vi "运维调试_总磷总氮.vi"() -> ()   [LabVIEW 2016, in "斯坦道CODcr.lvlib"]
uses:
  <vilib>/Utility/miscctls.llb/LVPointTypeDef.ctl
  <vilib>/Plasmionique/MB Master/MB_Master/MB_Master.lvclass
  <vilib>/ptbypt/NI_PtbyPt.lvlib
panel:
  out "seconds since 1Jan1904 2":timestamp
  out "seconds since 1Jan1904":timestamp
  in  "周期设置":bool
  in  "流程操作":bool
  out "消解压力":sgl format="%#.2f kPa"
  out "权限等级":string
  out "总步数":i32
  out "滑动杆":u8(slide) caption="测试进度" scale=0.0..100.0
  out "试剂余量显示":sgl[][](graph)
  in  "仪器校准":bool
  in  "参数查询":bool
  out "简易步骤名称":string
  in  "温度曲线":bool
  in  "试剂余量":bool
  in  "灯值调整":bool
  out "固件版本号":string
  out "模块版本号":string
  out "注射器温度":sgl format="%#.2f ℃"
  out "消解温度":sgl format="%#.2f ℃"
  out "ADC":sgl
  out "F3":sgl format="%#.6f"
  out "F2":sgl format="%#.6f"
  out "F1":sgl format="%#.6f"
  out "F0":sgl format="%#.6f"
  out "运行状态":T1 {"数据时间:" format="%<%y/%m/%d %H:%M:%S>T"; "仪器时间:" format="%<%y/%m/%d %H:%M:%S>T"}
  in  "单选按钮":T2=enum."总氮"
  in  "布尔":bool
  in  "外设固件":bool
  out "字符串 2":string
  in  "数组":string[](array[string])
  in  "返回":bool
  in  "参数设置":bool
  out "集成报警信息":string
  in  "停止":bool
  in  "手动启动":bool
  in  "调试":bool
  out "多列列表框":i32(listbox)
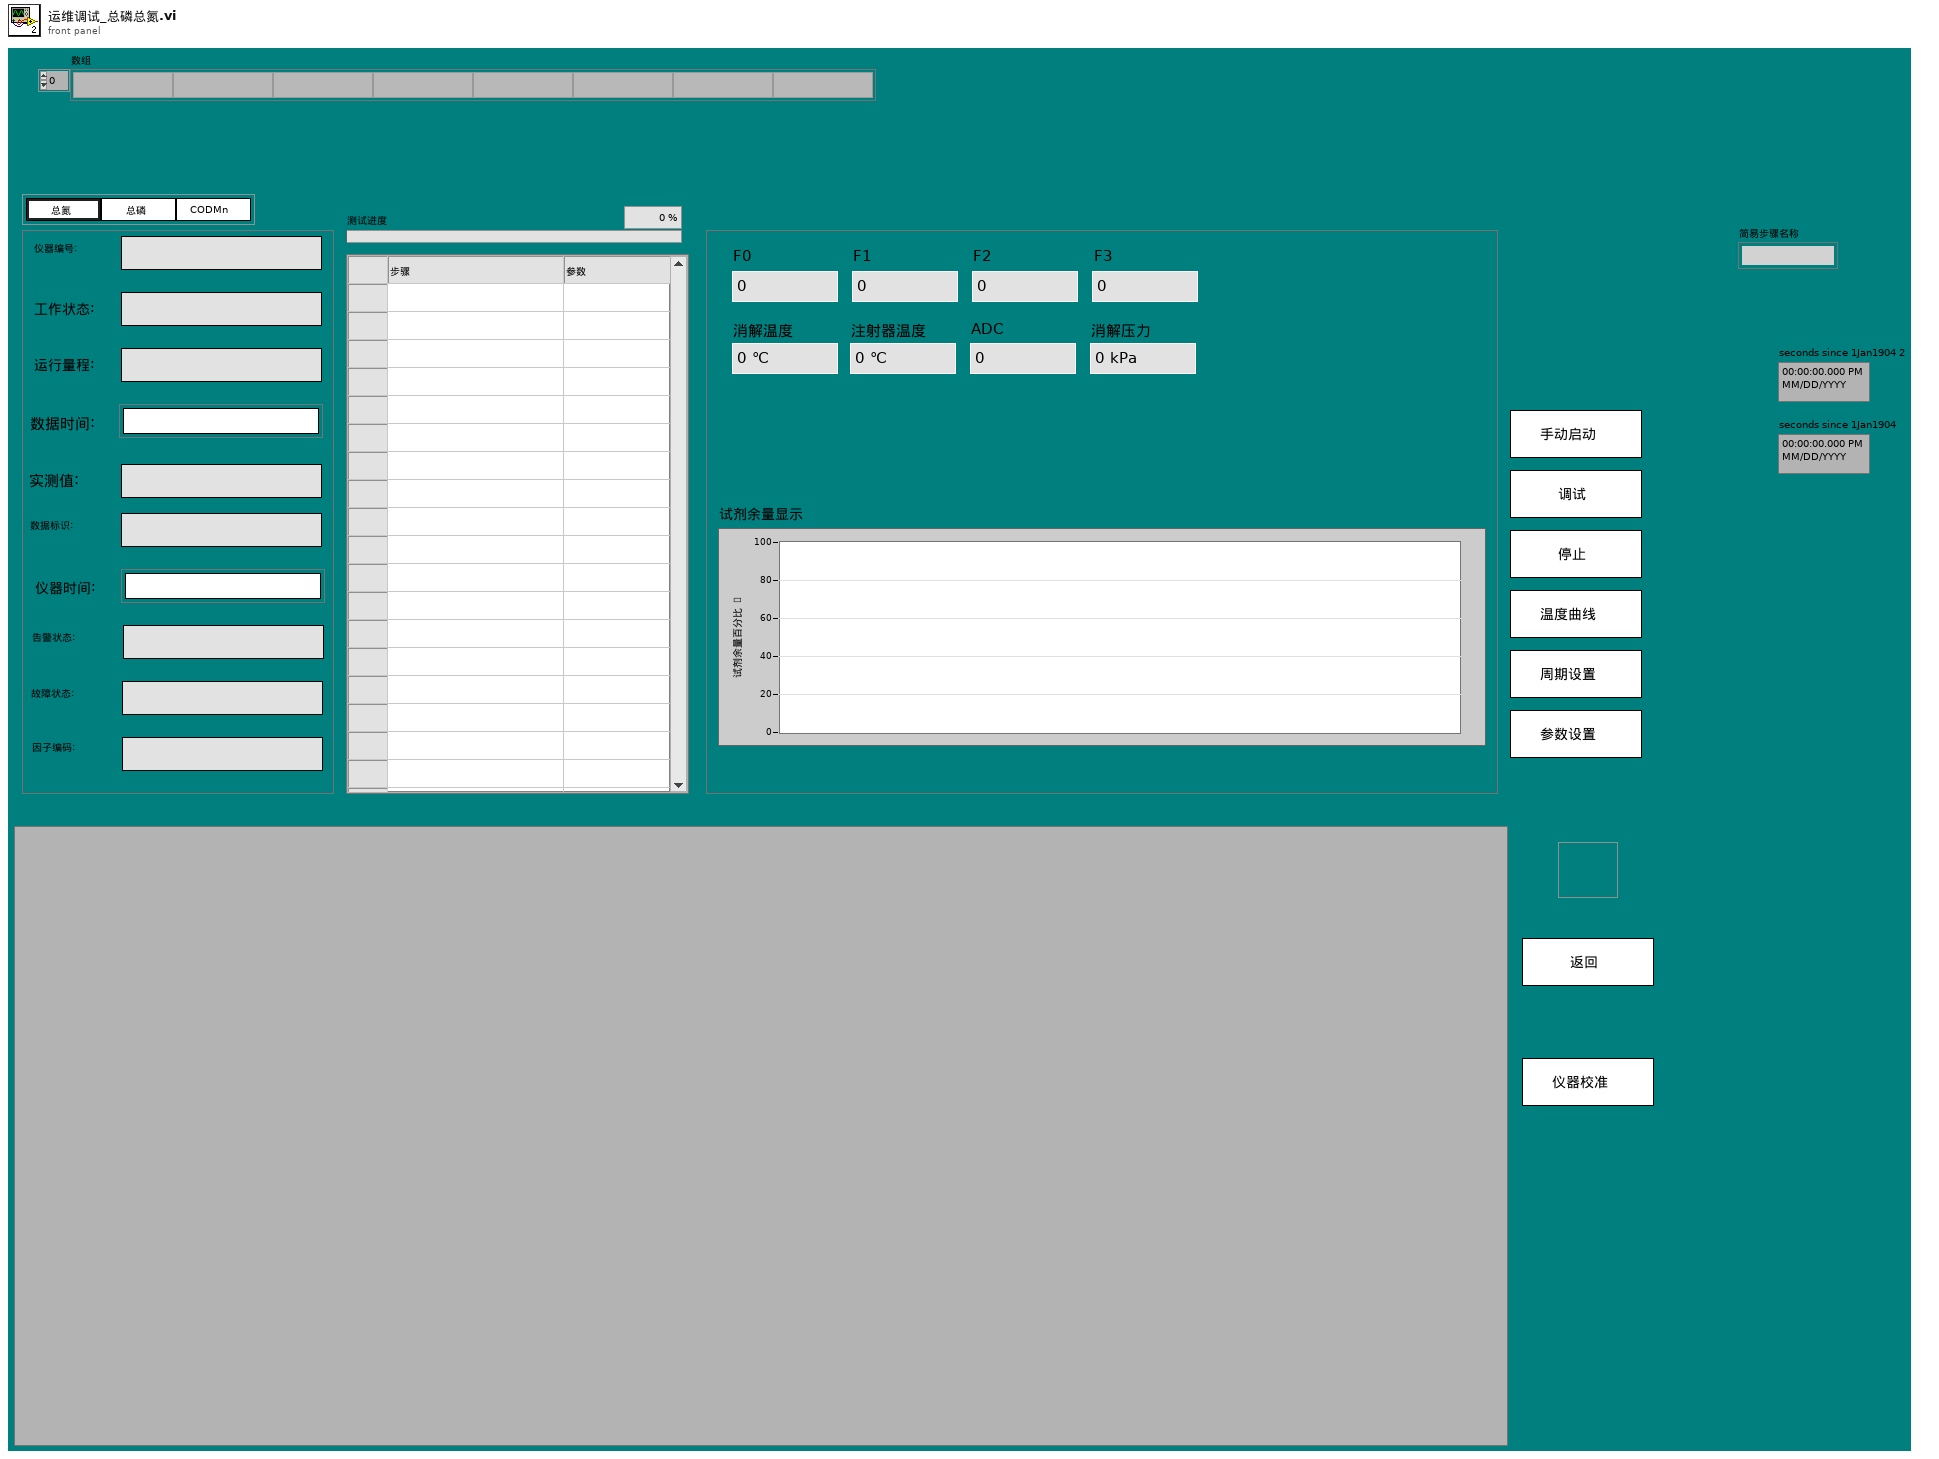
[diagram p1: front panel]
types:
  T1 = cluster{"仪器编号:":string, "工作状态:":string, "运行量程: ":string, "数据时间:":timestamp, "实测值:":string, "数据标识: ":string, "仪器时间:":timestamp, "告警状态: ":string, "故障状态:  ":string, "因子编码:":string}
  T2 = typedef "斯坦道CODcr.lvlib/启动参数显示控件.ctl" = enum32{"COD", "氨氮", "总氮", "总磷", "磷酸盐", "硝氮", "亚硝氮", "硅酸盐", "硫化物", "氟化物", "CODMn"}
  T3 = cluster{"Major":u16, "Minor":u16, "Fix":u16, "Build":u16}
  T4 = typedef "斯坦道总磷总氮.lvlib/启动参数显示控件.ctl" = enum32{"COD", "氨氮", "总氮", "总磷", "磷酸盐", "硝氮", "亚硝氮", "硅酸盐", "硫化物", "氟化物", "CODMn"}
  T5 = typedef "LVPointTypeDef.ctl" = cluster{"Horizontal":i16, "Vertical":i16}
  T6 = cluster{"系统时间":timestamp, "工作状态":u16, "测量模式":enum16{"待机", "连续模式", "周期模式", "定点模式", "受控模式", "手动模式"}, "告警代码":u16, "故障代码":u16, "日志代码":u16, "软件版本":u16, "F0":sgl, "F1":sgl, "F2":sgl, "F3":sgl, "T":sgl, "H":sgl, "id":u16, "flowid":u16, "量程":u16, "总磷控温温度1":sgl, "营养盐控温温度2":sgl, "ADC":sgl}
  T7 = cluster{"id":string, "ver":string, "type":string, "code":u16, "level":enum16{"一级", "二级", "三级"}, "message":string, "analysis":string, "platform_alarm_code":string}
  T8 = typedef "SingleStepTestV3.lvlib/SingleStepTestV3.lvclass/仪器版本.ctl" = enum16{"A版", "B版", "A1版"}
  T9 = cluster{"因子编码":u32, "单位":u16, "标样参考值":sgl, "水样数据时间":timestamp, "水样实测值":sgl, "水样数据标识":string, "标样数据时间":timestamp, "标样实测值":sgl, "标样数据标识":string, "空白数据时间":timestamp, "空白实测值":sgl, "空白数据标识":string, "零点核查数据时间":timestamp, "零点核查实测值":sgl, "零点核查数据标识":string, "跨度核查数据时间":timestamp, "跨度核查实测值":sgl, "跨度核查数据标识":string, "加标回收数据时间":timestamp, "加标回收实测值":sgl, "加标回收数据标识":string, "平行样数据时间":timestamp, "平行样实测值":sgl, "平行样数据标识":string, "F0":sgl, "F1":sgl, "F2":sgl, "F3":sgl, "F4":sgl, "F5":sgl, "F6":sgl, "F7":sgl, "温度":sgl, "湿度":sgl, "X值":sgl, "fidrange":u16, "X1值":sgl}[]
  T10 = cluster{"因子编码":u32, "单位":u16, "标样参考值":sgl, "水样数据时间":timestamp, "水样实测值":sgl, "水样数据标识":string, "标样数据时间":timestamp, "标样实测值":sgl, "标样数据标识":string, "空白数据时间":timestamp, "空白实测值":sgl, "空白数据标识":string, "零点核查数据时间":timestamp, "零点核查实测值":sgl, "零点核查数据标识":string, "跨度核查数据时间":timestamp, "跨度核查实测值":sgl, "跨度核查数据标识":string, "加标回收数据时间":timestamp, "加标回收实测值":sgl, "加标回收数据标识":string, "平行样数据时间":timestamp, "平行样实测值":sgl, "平行样数据标识":string, "F0":sgl, "F1":sgl, "F2":sgl, "F3":sgl, "F4":sgl, "F5":sgl, "F6":sgl, "F7":sgl, "温度":sgl, "湿度":sgl, "X值":sgl, "fidrange":u16, "X1值":sgl}
  T11 = typedef "报警信息字段定义.ctl" = cluster{"时间":timestamp, "参数":string, "报警信息":string, "备注":string, "code":u64, "platform_alarm_code":string, "报警标识":enum16{"产生", "消除"}}
  T12 = typedef "TimingControl.lvlib/TimingControl.lvclass/国标控制命令.ctl" = enum16{"启动测量", "标样核查", "零点核查", "跨度核查", "空白测试", "平行样测试", "加标回收", "空白校准", "标样校准", "初始化（清洗）", "停止测试", "仪器重启", "校时", "模式设置", "测量间隔设置"}
  T13 = typedef "TimingControl.lvlib/TimingControl.lvclass/测量参数.ctl" = u16
  T14 = enum32{"Bad", "Idle", "Run top level", "Running"}
  T15 = enum16{"空闲", "水样测试", "标样核查", "零点核查", "跨度核查", "空白测试", "平行样测试", "加标回收", "空白校准", "标样校准", "初始化（清洗）"}
  T16 = cluster{"站号":u16, "量程切换":enum32{"H", "L", "AUTO"}, "控制命令":enum16{"启动测量", "标样核查", "零点核查", "跨度核查", "空白测试", "平行样测试", "加标回收", "空白校准", "标样校准", "初始化（清洗）", "停止测试", "仪器重启", "校时", "模式设置", "测量间隔设置"}, "模式设置":enum16{"待机", "连续模式", "周期模式", "定点模式", "受控模式", "手动模式"}, "测量间隔":u16}
  T17 = cluster{"时间标识":timestamp, "设备":string, "日志信息":string, "流程参数":string}
  T18 = typedef "LVRowAndColumnUnsignedTypeDef.ctl" = cluster{"Row":u32, "Column":u32}
  T19 = typedef "操作日志字段定义.ctl" = cluster{"时间":timestamp, "参数":string, "日志信息":string, "流程参数":string}
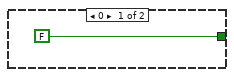
[diagram p4: hidden frame]
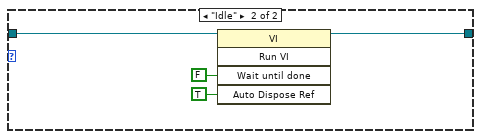
[diagram p8: hidden frame]
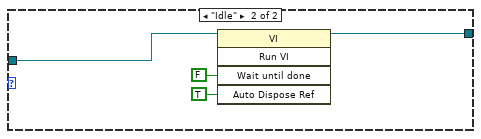
[diagram p9: hidden frame]
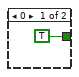
[diagram p11: hidden frame]
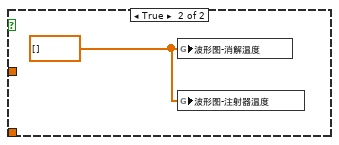
[diagram p12: hidden frame]
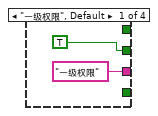
[diagram p18: hidden frame]
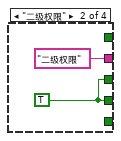
[diagram p19: hidden frame]
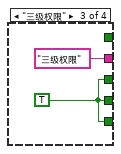
[diagram p20: hidden frame]
diagram:
  n1 = flat-sequence {
    tunnel: [w28] -> w18
    tunnel: w18 -> [w40]
    tunnel: [w40] -> w17
    tunnel: w17 -> [w65]
    tunnel: [w156] -> w19
    tunnel: [errorcluster {"status"=FALSE, "code"=0, "source"=""} ("错误输入（无错误）")] -> w8
    tunnel: [errorcluster {"status"=FALSE, "code"=0, "source"=""} ("错误输入（无错误）")] -> w7
    tunnel: [w153] -> w5
    tunnel: [errorcluster {"status"=FALSE, "code"=0, "source"=""} ("error out")] -> w4
    tunnel: [errorcluster {"status"=FALSE, "code"=0, "source"=""} ("错误输入（无错误）")] -> w3
    frame #0 {
      n2 = control-ref of="本VI"() -> (w30:refnum<vi>)
      n3 = control-ref of="本VI"() -> (w39:refnum<vi>)
      n4 = property class="VI"(reference=w30) -> ("Library"=w31:refnum<vi>)  [unwired: 1 in, 2 out]
      n5 = property class="VI"(reference=w39) -> ("Library.Version"=w38:T3)  [unwired: 1 in, 2 out]
      n6 = global read "VAR总磷总氮全局变量.vi" "初始化"() -> (w27:bool)
      n7 = case shown="假" w27 {
        frame False {
          n8 = call "配置初始化.vi"() -> ()  [unwired: 11 in, 1 out]
        }
        frame True {
        }
      }
      n9 = property class="Library"(reference=w31) -> ("Path"=w29:path)  [unwired: 1 in, 2 out]
      n10 = Unbundle By Name(w38) -> ("Major"=w36:u16, "Minor"=w35:u16, "Fix"=w34:u16, "Build"=w33:u16)
      n11 = call "新建通讯互斥锁.vi"() -> ()  [unwired: 11 in, 1 out]
      n12 = Format Into String(format string="模块版本号：%d.%d.%d.%d" ("格式字符串"), w36, w35, w34, w33) -> (resulting string=→"模块版本号":string)  [unwired: 2 in, 1 out]
      n13 = call <vilib>:"Get File Extension.vi"("file"=w29) -> ("filename without extension"=w28:string)  [unwired: 6 in, 4 out]
    }
    frame #1 {
      n14 = global read "总磷总氮断电保存全局变量.vi" "IP"() -> (w44:string)
      n15 = global read "总磷总氮断电保存全局变量.vi" "VISA Resource"() -> (w41:refnum<visa-resource-name>)
      n16 = Empty String/Path?(string/path=w44) -> (empty?=w43:bool)
      n17 = Empty String/Path?(string/path=w41) -> (empty?=w42:bool)
      n18 = case shown="真" w43 {
        tunnel: w40 -> [_ w56]
        frame False {
        }
        frame True {
          n19 = case shown="\"斯坦道CODMn\"" w56 {
            tunnel: [w57 "192.168.1.203" ("IP") "192.168.1.202" ("IP") "192.168.1.202" ("IP") "192.168.1.203" ("IP") "192.168.1.204" ("IP") "192.168.1.205" ("IP") "192.168.1.201" ("IP")] -> w55
            frame Default {
              n20 = global read "总磷总氮断电保存全局变量.vi" "IP"() -> (w57:string)
            }
            frame "斯坦道总磷总氮" {
            }
            frame "斯坦道氨氮" {
            }
            frame "斯坦道氨氮总磷" {
            }
            frame "斯坦道总磷" {
            }
            frame "斯坦道总氮" {
            }
            frame "斯坦道CODcr" {
            }
            frame "斯坦道CODMn" {
            }
          }
          n21 = global write "总磷总氮断电保存全局变量.vi" "IP"(w55) -> ()
        }
      }
      n22 = case shown="真" w42 {
        tunnel: w40 -> [_ w46]
        frame False {
        }
        frame True {
          n23 = case shown="\"斯坦道CODMn\"" w46 {
            tunnel: [w47 "COM5" ("IP") "COM7" ("IP") "COM7" ("IP") "COM5" ("IP") "COM10" ("IP") "COM9" ("IP") "COM4" ("IP")] -> w45
            frame Default {
              n24 = global read "总磷总氮断电保存全局变量.vi" "VISA Resource"() -> (w47:refnum<visa-resource-name>)
            }
            frame "斯坦道总磷总氮" {
            }
            frame "斯坦道氨氮" {
            }
            frame "斯坦道氨氮总磷" {
            }
            frame "斯坦道总磷" {
            }
            frame "斯坦道总氮" {
            }
            frame "斯坦道CODcr" {
            }
            frame "斯坦道CODMn" {
            }
          }
          n25 = global write "总磷总氮断电保存全局变量.vi" "VISA Resource"(w45) -> ()
        }
      }
    }
    frame #2 {
      n26 = global read "model config var.vi" "启动队列名称"() -> (w67:cluster{"String":string, "Value":u16}[])
      n27 = Empty Array?(array=w67) -> (empty?=w66:bool)
      n28 = case shown="真" w66 {
        tunnel: w65 -> [_ w68]
        frame False {
        }
        frame True {
          n29 = global read "总磷总氮断电保存全局变量.vi" "PORT"() -> (w74:string)
          n30 = Decimal String To Number(string=w74) -> (number=w73:i32)  [unwired: 2 in, 1 out]
          n31 = global read "总磷总氮断电保存全局变量.vi" "MB通信方式选择"() -> (w72:enum16{"串口", "TCP"})
          n32 = global read "总磷总氮断电保存全局变量.vi" "VISA Resource"() -> (w71:refnum<visa-resource-name>)
          n33 = global read "总磷总氮断电保存全局变量.vi" "IP"() -> (w75:string)
          n34 = call "获取启动参数.vi"("MB通信方式选择"=w72, "Port (502)"=w73, "IP Address"=w75, "VISA Resource"=w71) -> ("error out"=w70:errorcluster, "数组"=w69:cluster{"String":string, "Value":u16}[])  [unwired: 6 in]
          n35 = flat-sequence {
            tunnel: w70 -> [w77]
            tunnel: w69 -> [w76]
            tunnel: w68 -> [w79]
            frame #0 {
              n36 = case shown="无错误" w77 {
                tunnel: w76 -> [w78 _]
                frame No Error {
                  n37 = global write "model config var.vi" "启动队列名称"(w78) -> ()
                }
                frame Error {
                }
              }
            }
            frame #1 {
              n38 = global read "model config var.vi" "启动队列名称"() -> (w81:cluster{"String":string, "Value":u16}[])
              n39 = Empty Array?(array=w81) -> (empty?=w80:bool)
              n40 = case shown="真" w80 {
                tunnel: w79 -> [_ w82]
                frame False {
                }
                frame True {
                  n41 = case shown="\"斯坦道CODmn\"" w82 {
                    frame Default {
                    }
                    frame "斯坦道总磷总氮" {
                      n42 = global write "model config var.vi" "启动队列名称"(cluster{"String":string, "Value":u16}[] [{"String"="总氮", "Value"=2}, {"String"="总磷", "Value"=1}] ("启动队列名称")) -> ()
                    }
                    frame "斯坦道氨氮" {
                      n43 = global write "model config var.vi" "启动队列名称"(cluster{"String":string, "Value":u16}[] [{"String"="氨氮", "Value"=3}] ("启动队列名称")) -> ()
                    }
                    frame "斯坦道氨氮总磷" {
                      n44 = global write "model config var.vi" "启动队列名称"(cluster{"String":string, "Value":u16}[] [{"String"="氨氮", "Value"=3}, {"String"="总磷", "Value"=1}] ("启动队列名称")) -> ()
                    }
                    frame "斯坦道总磷" {
                      n45 = global write "model config var.vi" "启动队列名称"(cluster{"String":string, "Value":u16}[] [{"String"="总磷", "Value"=1}] ("启动队列名称")) -> ()
                    }
                    frame "斯坦道总氮" {
                      n46 = global write "model config var.vi" "启动队列名称"(cluster{"String":string, "Value":u16}[] [{"String"="总氮", "Value"=2}] ("启动队列名称")) -> ()
                    }
                    frame "斯坦道CODcr" {
                      n47 = global write "model config var.vi" "启动队列名称"(cluster{"String":string, "Value":u16}[] [{"String"="CODcr", "Value"=22}] ("启动队列名称")) -> ()
                    }
                    frame "斯坦道氟化物" {
                      n48 = global write "model config var.vi" "启动队列名称"(cluster{"String":string, "Value":u16}[] [{"String"="氟化物", "Value"=50}] ("启动队列名称")) -> ()
                    }
                    frame "斯坦道CODmn" {
                      n49 = global write "model config var.vi" "启动队列名称"(cluster{"String":string, "Value":u16}[] [{"String"="CODMn", "Value"=21}] ("启动队列名称")) -> ()
                    }
                  }
                }
              }
            }
            frame #2 {
              n50 = call "模块配置写入.vi"() -> ()  [unwired: 11 in, 1 out]
            }
          }
        }
      }
    }
    frame #3 {
      # "初始化"
      n51 = global read "总磷总氮断电保存全局变量.vi" "流程路径"() -> (w95:path)
      n52 = global read "model config var.vi" "启动队列名称"() -> (w101:cluster{"String":string, "Value":u16}[])
      n53 = global read "总磷总氮断电保存全局变量.vi" "简易流程路径"() -> (w92:path)
      n54 = call <vilib>:"Check if File or Folder Exists.vi"("path"=w95) -> ("file or folder exists?"=w100:bool)  [unwired: 8 in, 2 out]
      n55 = for {
        tunnel: w101 -> [w118] mode=indexing
        shift-right: [w117] -> w102
        shift-left: "" -> [w115]
        n56 = Unbundle By Name(w118) -> ("String"=w116:string)
        n57 = Concatenate Strings(w115, w116) -> (w117:string)
      }
      n58 = call <vilib>:"Check if File or Folder Exists.vi"("path"=w92) -> ("file or folder exists?"=w99:bool)  [unwired: 8 in, 2 out]
      n59 = Empty String/Path?(string/path=w95) -> (empty?=w96:bool)
      n60 = Not(x=w100) -> (.not. x?=w98:bool)
      n61 = Empty String/Path?(string/path=w92) -> (empty?=w91:bool)
      n62 = Not(x=w99) -> (.not. x?=w94:bool)
      n63 = Or(x=w96, y=w98) -> (x .or. y?=w97:bool)
      n64 = Or(x=w91, y=w94) -> (x .or. y?=w93:bool)
      n65 = case shown="真" w97 {
        frame False {
        }
        frame True {
          n66 = global read "model config var.vi" "启动队列名称"() -> (w111:cluster{"String":string, "Value":u16}[])
          n67 = for {
            tunnel: w111 -> [w114] mode=indexing
            tunnel: [w113] -> w110 mode=indexing
            n68 = Unbundle By Name(w114) -> ("String"=w113:string)
          }
          n69 = call "获取默认流程路径.vi"("参数"=w110) -> ("路径"=w112:path)  [unwired: 10 in]
          n70 = global write "总磷总氮断电保存全局变量.vi" "流程路径"(w112) -> ()
        }
      }
      n71 = case shown="真" w93 {
        frame False {
        }
        frame True {
          n72 = global read "model config var.vi" "启动队列名称"() -> (w106:cluster{"String":string, "Value":u16}[])
          n73 = for {
            tunnel: w106 -> [w109] mode=indexing
            tunnel: [w108] -> w105 mode=indexing
            n74 = Unbundle By Name(w109) -> ("String"=w108:string)
          }
          n75 = call "获取默认流程路径.vi"("复合步骤"=TRUE, "参数"=w105) -> ("路径"=w107:path)  [unwired: 9 in]
          n76 = global write "总磷总氮断电保存全局变量.vi" "简易流程路径"(w107) -> ()
        }
      }
      n77 = global write "VAR总磷总氮全局变量.vi" "模块名称"(w102) -> ()
    }
    frame #4 {
      n78 = global read "model config var.vi" "启动队列名称"() -> (w121:cluster{"String":string, "Value":u16}[])
      n79 = vi-ref "总磷总氮测量数据储存.vi"() -> (w131:refnum<vi>)
      n80 = vi-ref "总磷总氮通讯.vi"() -> (w123:refnum<vi>)
      n81 = Index Array(array=w121) -> (element=w120:cluster{"String":string, "Value":u16})  [unwired: 1 in]
      n82 = property class="VI"(reference=w131) -> ("Name"=w138:string)  [unwired: 1 in, 2 out]
      n83 = property class="VI"(reference=w123) -> ("Name"=w124:string)  [unwired: 1 in, 2 out]
      n84 = Unbundle By Name(w120) -> ("Value"=w119:u16)
      n85 = case shown="50" w119 {
        tunnel: [w139 启动参数显示控件."总磷" ("单选按钮") 启动参数显示控件."总氮" ("单选按钮") 启动参数显示控件."COD" ("单选按钮") 启动参数显示控件."氨氮" ("单选按钮") 启动参数显示控件."磷酸盐" ("单选按钮") 启动参数显示控件."硝氮" ("单选按钮") 启动参数显示控件."亚硝氮" ("单选按钮") 启动参数显示控件."硅酸盐" ("单选按钮") 启动参数显示控件."硫化物" ("单选按钮") 启动参数显示控件."氟化物" ("单选按钮") 启动参数显示控件."CODMn" ("单选按钮")] -> w122
        frame 0, Default {
          n86 = property on="单选按钮" class="RadioBtnsControl (严格)"() -> ("Value"=w139:T4)  [unwired: 2 in, 2 out]
        }
        frame 1 {
        }
        frame 2 {
        }
        frame 22 {
        }
        frame 3 {
        }
        frame 4 {
        }
        frame 5 {
        }
        frame 6 {
        }
        frame 7 {
        }
        frame 8 {
        }
        frame 50 {
        }
        frame 21 {
        }
      }
      n87 = Open VI Reference(type specifier VI Refnum (for type only)=refnum<vi> refnum, vi path=w138, options=128 ("选项")) -> (vi reference=w136:refnum<vi>, error out=w134:errorcluster)  [unwired: 3 in]
      n88 = Open VI Reference(type specifier VI Refnum (for type only)=refnum<vi> refnum, vi path=w124, options=128 ("选项")) -> (vi reference=w126:refnum<vi>, error out=w128:errorcluster)  [unwired: 3 in]
      n89 = call-by-ref "开始异步调用"(reference=w136, error in=w134) -> (reference out=w132:refnum<vi>, error out=w133:errorcluster)  [unwired: 12 in]
      n90 = call-by-ref "开始异步调用"(reference=w126, error in=w128) -> (reference out=w130:refnum<vi>, error out=w129:errorcluster)  [unwired: 12 in]
      n91 = Close Reference(reference=w132, error in (no error)=w133) -> ()  [unwired: 1 out]
      n92 = Close Reference(reference=w130, error in (no error)=w129) -> ()  [unwired: 1 out]
      n93 = property on="单选按钮" class="RadioBtnsControl (严格)"("Value"=w122) -> ()  [unwired: 2 in, 2 out]
    }
    frame #5 {
      n94 = call "配置文件路径.vi"() -> ("appended path"=w153:path)  [unwired: 11 in]
      n95 = call "设置模块队列名.vi"() -> ("Msg"=w156:string)  [unwired: 5 in]
    }
  }
  n96 = flat-sequence {
    frame #0 {
      n97 = property on="窗格" class="Pane"("Origin"=T5 {"Horizontal"=0, "Vertical"=0} ("原点")) -> ()  [unwired: 2 in, 2 out]
    }
  }
  n98 = call "Create balloon 队列.vi"() -> ("队列输出"=w23:refnum<queue>)  [unwired: 11 in]
  n99 = while {
    stop <- FALSE stop-if-true
    n100 = global read "VAR总磷总氮全局变量.vi" "状态告警区"() -> (w162:T6)
    n101 = Unbundle By Name(w162) -> ("工作状态"=w160:u16)
    n102 = Equal To 0?(x=w160) -> (x = 0?=w159:bool)
    n103 = global read "VAR总磷总氮全局变量.vi" "通讯状态"() -> (w163:bool)
    n104 = And(x=w159, y=w163) -> (x .and. y?=w161:bool)
    n105 = call <vilib>:"Boolean Crossing PtByPt.vi"("input"=w161) -> ("crossing"=w158:bool)  [unwired: 2 in]
    n106 = case shown="真" w158 {
      frame False {
      }
      frame True {
        n107 = control-ref of="试剂余量显示"() -> (w166:refnum<vi>)
        n108 = call "试剂余量展示.vi"("波形图 2"=w166) -> ("波形图"=→"试剂余量显示":sgl[][])  [unwired: 10 in]
      }
    }
    n109 = Wait (ms)(milliseconds to wait=u32 1000 ("等待时间（毫秒）")) -> ()  [unwired: 1 out]
  }
  n110 = while {
    shift-right: [w177] -> _
    shift-left: u32 0 ("y") -> [w179]
    stop <- FALSE stop-if-true
    # "密码权限"
    n111 = global read "VAR总磷总氮全局变量.vi" "权限等级"() -> (w174:enum16{"一级权限", "二级权限", "三级权限", "超级权限"})
    n112 = case shown="\"超级权限\"" w174 {
      tunnel: [_ w184 w186 w189] -> w168
      tunnel: [_ _ w186 w189] -> _
      tunnel: [_ w184 w186 w189] -> w173
      tunnel: [_ _ _ TRUE] -> _
      tunnel: [TRUE _ _ _] -> w171
      tunnel: ["一级权限" "二级权限" "三级权限" "超级权限"] -> w169
      frame "一级权限", Default {
      }
      frame "二级权限" {
        w184 = TRUE
      }
      frame "三级权限" {
        w186 = TRUE
      }
      frame "超级权限" {
        w189 = TRUE
      }
    }
    "权限等级" <- w169
    n113 = case shown="假" "布尔" {
      tunnel: w179 -> [_ w192]
      tunnel: [_ w191] -> w177
      frame False {
      }
      frame True {
        n114 = Increment(x=w192) -> (x+1=w191:u32)
      }
    }
    n115 = Wait (ms)(milliseconds to wait=u32 1000 ("等待时间（毫秒）")) -> ()  [unwired: 1 out]
    n116 = Not(x=w171) -> (.not. x?=w170:bool)
    n117 = property on="外设固件" class="Bool"("Visible"=w173) -> ()  [unwired: 2 in, 2 out]
    n118 = property on="流程操作" class="Bool"("Visible"=w168) -> ()  [unwired: 2 in, 2 out]
    n119 = property on="试剂余量" class="Bool"("Visible"=w168) -> ()  [unwired: 2 in, 2 out]
    n120 = property on="灯值调整" class="Bool"("Visible"=w168) -> ()  [unwired: 2 in, 2 out]
    n121 = Greater Or Equal?(x=w177, y=u32 3600) -> (x >= y?=w175:bool)
    n122 = property on="布尔" class="Bool (严格)"("Value"=w170) -> ()  [unwired: 2 in, 2 out]
    n123 = case shown="真" w175 {
      frame False {
      }
      frame True {
        n124 = global write "VAR总磷总氮全局变量.vi" "权限等级"(enum16{"一级权限", "二级权限", "三级权限", "超级权限"}."一级权限" ("权限等级")) -> ()
      }
    }
  }
  n125 = while {
    shift-right: [w203] -> _
    shift-left: u16 1 ("工作状态") -> [w201]
    stop <- FALSE stop-if-true
    (unwired) "注射器温度"
    n126 = global read "VAR总磷总氮全局变量.vi" "状态告警区"() -> (w224:T6)
    n127 = global read "VAR总磷总氮全局变量.vi" "通讯状态"() -> (w235:bool)
    n128 = global read "VAR总磷总氮全局变量.vi" "状态告警区"() -> (w233:T6)
    n129 = global write "VAR总磷总氮全局变量.vi" "最近一次工作状态"(w201) -> ()
    n130 = Unbundle By Name(w224) -> ("id"=w223:u16, "工作状态"=w219:u16)
    n131 = case shown="真" w235 {
      tunnel: ["通讯异常" ("集成报警信息") w354] -> w234
      frame False {
      }
      frame True {
        n132 = global read "VAR总磷总氮全局变量.vi" "状态告警区"() -> (w356:T6)
        n133 = local read "seconds since 1Jan1904 2"() -> (w346:timestamp)
        n134 = local read "seconds since 1Jan1904"() -> (w349:timestamp)
        n135 = Subtract(x=w346, y=w349) -> (x-y=w345:dbl)
        n136 = Unbundle By Name(w356) -> ("工作状态"=w352:u16)
        n137 = Not Equal To 0?(x=w352) -> (x != 0?=w348:bool)
        n138 = Get Date/Time In Seconds() -> (seconds since 1Jan1904=w347:timestamp)
        n139 = global read "VAR总磷总氮全局变量.vi" "测量状态"() -> (w353:string)
        n140 = Greater Or Equal?(x=w345, y=36000.0) -> (x >= y?=w342:bool)
        n141 = case shown="真" w348 {
          tunnel: w347 -> [_ w357]
          frame False {
          }
          frame True {
            "seconds since 1Jan1904 2" <- w357
          }
        }
        n142 = Format Into String(format string="工作计时: %d 秒" ("格式字符串"), initial string=w353, w345) -> (resulting string=w354:string)  [unwired: 1 in, 1 out]
        n143 = call <vilib>:"Boolean Crossing PtByPt.vi"("direction"=enum16{"either", "false-true", "true-false"}."false-true", "input"=w348) -> ("crossing"=w350:bool)  [unwired: 1 in]
        n144 = Or(x=w350, y=w342) -> (x .or. y?=w343:bool)
        n145 = case shown="真" w343 {
          tunnel: w347 -> [_ w358]
          frame False {
          }
          frame True {
            "seconds since 1Jan1904" <- w358
          }
        }
      }
    }
    "集成报警信息" <- w234
    n146 = Unbundle By Name(w233) -> ("flowid"=w200:u16, "系统时间"=w229:timestamp, "工作状态"=w228:u16, "告警代码"=w222:u16, "故障代码"=w221:u16, "量程"=w227:u16)
    n147 = case shown="\"磷酸盐\"" "单选按钮" {
      tunnel: [22 3 2 1 4 5 6 7 8 50 21] -> w204
      tunnel: [_ TRUE _ _ _ _ _ _ _ _ _] -> w195
      frame "COD", Default {
      }
      frame "氨氮" {
      }
      frame "总氮" {
      }
      frame "总磷" {
      }
      frame "磷酸盐" {
      }
      frame "硝氮" {
      }
      frame "亚硝氮" {
      }
      frame "硅酸盐" {
      }
      frame "硫化物" {
      }
      frame "氟化物" {
      }
      frame "CODMn" {
      }
    }
    n148 = case shown="1, 默认" w219 {
      tunnel: w223 -> [_ w291]
      frame 0 {
      }
      frame 1, Default {
        n149 = case shown="21" w291 {
          tunnel: [w292 启动参数显示控件."总磷" ("单选按钮") 启动参数显示控件."总氮" ("单选按钮") 启动参数显示控件."COD" ("单选按钮") 启动参数显示控件."氨氮" ("单选按钮") 启动参数显示控件."磷酸盐" ("单选按钮") 启动参数显示控件."硝氮" ("单选按钮") 启动参数显示控件."亚硝氮" ("单选按钮") 启动参数显示控件."硅酸盐" ("单选按钮") 启动参数显示控件."硫化物" ("单选按钮") 启动参数显示控件."CODMn" ("单选按钮") 启动参数显示控件."氟化物" ("单选按钮")] -> w290
          frame 0, Default {
            n150 = property on="单选按钮" class="RadioBtnsControl (严格)"() -> ("Value"=w292:T4)  [unwired: 2 in, 2 out]
          }
          frame 1 {
          }
          frame 2 {
          }
          frame 22 {
          }
          frame 3 {
          }
          frame 4 {
          }
          frame 5 {
          }
          frame 6 {
          }
          frame 7 {
          }
          frame 8 {
          }
          frame 21 {
          }
          frame 50 {
          }
        }
        n151 = property on="单选按钮" class="RadioBtnsControl (严格)"("Value"=w290) -> ()  [unwired: 2 in, 2 out]
      }
    }
    n152 = case shown="2" w228 {
      selector: w228 -> [w308 _ w314 w318 w321 w323 w325 w327 w329 w331 w333 w335 w337 w340]
      tunnel: [w309 "空闲" ("工作状态") "水样测量" ("工作状态") w317 "零点核查" ("工作状态") "跨度核查" ("工作状态") "空白测试" ("工作状态") "平行样测试" ("工作状态") "加标回收" ("工作状态") "空白校准" ("工作状态") "标样校准" ("工作状态") "初始化" ("工作状态") "单步调试" ("工作状态") w339] -> w202
      tunnel: [w307 w312 w314 w318 w321 w323 w325 w327 w329 w331 w333 w335 w337 w340] -> w203
      tunnel: w201 -> [w307 w312 _ _ _ _ _ _ _ _ _ _ _ _]
      tunnel: w200 -> [_ _ _ w316 _ _ _ _ _ _ _ _ _ _]
      frame Default {
        n153 = Format Into String(format string="%d" ("格式字符串"), initial string="未知" ("工作状态"), w308) -> (resulting string=w309:string)  [unwired: 1 in, 1 out]
      }
      frame 0 {
      }
      frame 1 {
      }
      frame 2 {
        n154 = case shown="5" w316 {
          tunnel: ["标样核查" ("工作状态") "快捷测试" ("工作状态")] -> w317
          frame 0, Default {
          }
          frame 5 {
          }
        }
      }
      frame 3 {
      }
      frame 4 {
      }
      frame 5 {
      }
      frame 6 {
      }
      frame 7 {
      }
      frame 8 {
      }
      frame 9 {
      }
      frame 10 {
      }
      frame 254 {
      }
      frame 255 {
        n155 = local read "简易步骤名称"() -> (w339:string)
      }
    }
    n156 = call "告警码字段定义.vi"("告警代码"=w222) -> ("告警信息"=w199:T7)  [unwired: 10 in]
    n157 = call "故障码字段定义.vi"("故障代码"=w221) -> ("告警信息"=w220:T7)  [unwired: 10 in]
    n158 = case shown="1" w227 {
      tunnel: ["" ("字符串") "低量程 " ("字符串") "高量程 " ("字符串")] -> w226
      frame Default {
      }
      frame 0 {
      }
      frame 1 {
      }
    }
    n159 = Unbundle By Name(w199) -> ("message"=w198:string)
    n160 = Unbundle By Name(w220) -> ("message"=w193:string)
    n161 = call "id参数转换.vi"("id"=w204) -> ("数组资源索引"=w205:i32)  [unwired: 9 in, 1 out]
    n162 = call "版本判断.vi"() -> ("仪器版本"=w197:T8)  [unwired: 11 in]
    n163 = global read "VAR总磷总氮全局变量.vi" "测量数据区数组"() -> (w208:T9)
    n164 = case shown="\"A版\", 默认" w197 {
      tunnel: [w238 "传感器" ("标题.文本")] -> w194
      tunnel: ["%#.2f ℃" ("数值文本.格式字符串") "%#.2f " ("数值文本.格式字符串")] -> w196
      tunnel: w195 -> [w241 _]
      frame "A版", Default {
        n165 = Select(t="显色温度", s=w241, f="注射器温度" ("标题.文本")) -> (s? t:f=w238:string)
      }
      frame "B版" {
      }
    }
    n166 = Index Array(array=w208, index=w205) -> (element=w207:T10)
    n167 = case shown="0, 默认" w201 {
      tunnel: [w259 w265 w269 w273 w277 w281 w285 w289] -> w218
      tunnel: [w257 w264 w268 w272 w275 w280 w284 w288] -> w213
      tunnel: [w260 w263 w267 w271 w274 w279 w283 w287] -> w211
      tunnel: w207 -> [_ w262 w266 w270 w276 w278 w282 w286]
      frame 0, Default {
        n168 = local read "运行状态"() -> (w261:T1)
        n169 = Unbundle By Name(w261) -> ("数据时间:"=w259:timestamp, "实测值:"=w258:string, "数据标识:"=w260:string)
        n170 = Fract/Exp String To Number(string=w258) -> (number=w257:dbl)  [unwired: 3 in, 1 out]
      }
      frame 1 {
        n171 = Unbundle By Name(w262) -> ("水样数据时间"=w265:timestamp, "水样实测值"=w264:sgl, "水样数据标识"=w263:string)
      }
      frame 2, 9 {
        n172 = Unbundle By Name(w266) -> ("标样数据时间"=w269:timestamp, "标样实测值"=w268:sgl, "标样数据标识"=w267:string)
      }
      frame 3 {
        n173 = Unbundle By Name(w270) -> ("零点核查数据时间"=w273:timestamp, "零点核查实测值"=w272:sgl, "零点核查数据标识"=w271:string)
      }
      frame 4 {
        n174 = Unbundle By Name(w276) -> ("跨度核查数据时间"=w277:timestamp, "跨度核查实测值"=w275:sgl, "跨度核查数据标识"=w274:string)
      }
      frame 7 {
        n175 = Unbundle By Name(w278) -> ("加标回收数据时间"=w281:timestamp, "加标回收实测值"=w280:sgl, "加标回收数据标识"=w279:string)
      }
      frame 5, 8 {
        n176 = Unbundle By Name(w282) -> ("空白数据时间"=w285:timestamp, "空白实测值"=w284:sgl, "空白数据标识"=w283:string)
      }
      frame 6 {
        n177 = Unbundle By Name(w286) -> ("平行样数据时间"=w289:timestamp, "平行样实测值"=w288:sgl, "平行样数据标识"=w287:string)
      }
    }
    n178 = Unbundle By Name(w207) -> ("因子编码"=w209:u32)
    n179 = global write "VAR总磷总氮全局变量.vi" "工作状态:"(w202) -> ()
    n180 = Format Into String(format string="w%05d" ("格式字符串"), w209) -> (resulting string=w225:string)  [unwired: 2 in, 1 out]
    n181 = property on="注射器温度" class="DigNum (严格)"("Caption.Text"=w194, "NumText.FormatString"=w196) -> ()  [unwired: 2 in, 2 out]
    n182 = Wait (ms)(milliseconds to wait=u32 1000 ("等待时间（毫秒）")) -> ()  [unwired: 1 out]
    n183 = Number To Fractional String(number=w213, precision (6)=i16 4 ("精度(6)")) -> (F-format string=w215:string)  [unwired: 2 in]
    n184 = Concatenate Strings(w215, " " ("字符串"), "mg/L" ("字符串")) -> (w212:string)
    n185 = global read "VAR总磷总氮全局变量.vi" "序列号"() -> (w230:string)
    n186 = Bundle By Name(cluster=T1 {"仪器编号:"="", "工作状态:"="", "运行量程: "="", "数据时间:"=timestamp(0 s since 1904-01-01), "实测值:"="", "数据标识: "="", "仪器时间:"=timestamp(0 s since 1904-01-01), "告警状态: "="", "故障状态:  "="", "因子编码:"=""} ("运行状态"), "仪器编号:"=w230, "仪器时间:"=w229, "工作状态:"=w202, "告警状态:"=w198, "故障状态:"=w193, "运行量程:"=w226, "数据时间:"=w218, "实测值:"=w212, "数据标识:"=w211, "因子编码:"=w225) -> (→"运行状态":T1)
  }
  n187 = while {
    shift-right: [w363] -> _
    shift-left: 0 -> [w364]
    stop <- FALSE stop-if-true
    n188 = global read "VAR总磷总氮全局变量.vi" "心跳包打开状态"() -> (w359:bool)
    n189 = case shown="假" w359 {
      tunnel: w364 -> [w368 _]
      tunnel: [w367 _] -> w363
      frame False {
        n190 = Increment(x=w368) -> (x+1=w367:i32)
      }
      frame True {
      }
    }
    n191 = Wait (ms)(milliseconds to wait=u32 1000 ("等待时间（毫秒）")) -> ()  [unwired: 1 out]
    n192 = Greater Or Equal?(x=w363, y=600) -> (x >= y?=w361:bool)
    n193 = case shown="真" w361 {
      frame False {
      }
      frame True {
        n194 = global write "VAR总磷总氮全局变量.vi" "升级固件关闭心跳包"(FALSE ("关闭心跳包")) -> ()
      }
    }
  }
  n195 = while {
    shift-right: [w370] -> _
    shift-left: TRUE -> [w371]
    stop <- FALSE stop-if-true
    n196 = global read "VAR总磷总氮全局变量.vi" "状态告警区"() -> (w374:T6)
    n197 = global read "VAR总磷总氮全局变量.vi" "状态告警区"() -> (w377:T6)
    n198 = Unbundle By Name(w374) -> ("总磷控温温度1"=w373:sgl)
    n199 = Unbundle By Name(w377) -> ("工作状态"=w372:u16, "总磷控温温度1"=w376:sgl, "营养盐控温温度2"=w375:sgl)
    n200 = call "消解压力计算.vi"("当前消解温度"=w373) -> ("消解压力"=→"消解压力":dbl)  [unwired: 10 in]
    n201 = case shown="1, 默认" w372 {
      tunnel: w376 -> [_ w383]
      tunnel: w375 -> [_ w382]
      tunnel: w371 -> [_ w381]
      tunnel: [TRUE _] -> w370
      frame 0 {
      }
      frame 1, Default {
        n202 = case shown="假" w381 {
          tunnel: w383 -> [w389 _]
          tunnel: w382 -> [w388 _]
          frame False {
            n203 = global read "VAR总磷总氮全局变量.vi" "波形图-消解温度"() -> (w387:sgl[])
            n204 = global read "VAR总磷总氮全局变量.vi" "波形图-注射器温度"() -> (w386:sgl[])
            n205 = Build Array (concatenate)(w387, w389) -> (w385:sgl[])
            n206 = Build Array (concatenate)(w386, w388) -> (w384:sgl[])
            n207 = global write "VAR总磷总氮全局变量.vi" "波形图-消解温度"(w385) -> ()
            n208 = global write "VAR总磷总氮全局变量.vi" "波形图-注射器温度"(w384) -> ()
          }
          frame True {
            w390 = dbl[] [] ("波形图-消解温度")
            n209 = global write "VAR总磷总氮全局变量.vi" "波形图-消解温度"(w390) -> ()
            n210 = global write "VAR总磷总氮全局变量.vi" "波形图-注射器温度"(w390) -> ()
          }
        }
      }
    }
    n211 = Wait (ms)(milliseconds to wait=u32 1000 ("等待时间（毫秒）")) -> ()  [unwired: 1 out]
  }
  n212 = while {
    tunnel: w23 -> [w397]
    shift-right: [w393] -> _
    shift-left: _ -> [w394]
    stop <- FALSE stop-if-true
    n213 = global read "VAR总磷总氮全局变量.vi" "状态告警区"() -> (w391:T6)
    n214 = Unbundle By Name(w391) -> ("工作状态"=w392:u16, "id"=w399:u16, "日志代码"=w398:u16, "故障代码"=w396:u16, "告警代码"=w395:u16)
    n215 = case shown="1, 默认" w392 {
      tunnel: w399 -> [_ _]
      tunnel: w398 -> [_ w411]
      tunnel: w397 -> [_ w410]
      tunnel: w396 -> [_ w409]
      tunnel: w395 -> [_ w408]
      tunnel: w394 -> [w402 w407]
      tunnel: [w402 w406] -> w393
      frame 0 {
      }
      frame 1, Default {
        n216 = Add(x=w409, y=w408) -> (x+y=w406:u16)
        n217 = Not Equal To 0?(x=w406) -> (x != 0?=w405:bool)
        n218 = Not Equal?(x=w406, y=w407) -> (x != y?=w404:bool)
        n219 = And(x=w405, y=w404) -> (x .and. y?=w403:bool)
        n220 = case shown="真" w403 {
          tunnel: w411 -> [_ w421]
          tunnel: w410 -> [_ w420]
          tunnel: w409 -> [_ w416]
          tunnel: w408 -> [_ w414]
          frame False {
          }
          frame True {
            n221 = Not Equal To 0?(x=w416) -> (x != 0?=w412:bool)
            n222 = global read "VAR总磷总氮全局变量.vi" "模块名称"() -> (w419:string)
            n223 = Not Equal To 0?(x=w414) -> (x != 0?=w413:bool)
            n224 = call "故障告警分析.vi"("告警代码"=w414, "故障代码"=w416, "运行步序"=w421, "参数"=w419) -> ("告警记录"=w415:T11, "故障记录"=w418:T11, "简易报警状态"=w417:cluster{"故障状态":string, "报警状态":string})  [unwired: 5 in]
            n225 = call "balloon入队列.vi"("报警内容"=w417, "队列"=w420) -> ()  [unwired: 9 in, 1 out]
            n226 = case shown="真" w412 {
              tunnel: w418 -> [_ w422]
              frame False {
              }
              frame True {
                n227 = call "总磷总氮报警信息.vi"("data in"=w422) -> ()  [unwired: 10 in, 1 out]
              }
            }
            n228 = case shown="真" w413 {
              tunnel: w415 -> [_ w423]
              frame False {
              }
              frame True {
                n229 = call "总磷总氮报警信息.vi"("data in"=w423) -> ()  [unwired: 10 in, 1 out]
              }
            }
          }
        }
      }
    }
    n230 = Wait (ms)(milliseconds to wait=u32 100) -> ()  [unwired: 1 out]
  }
  n231 = while {
    shift-right: [w424] -> _
    shift-left: _ -> [w429]
    tunnel: w5 -> [w427]
    stop <- FALSE stop-if-true
    n232 = File/Directory Info(path=w427) -> (last mod=w424:timestamp, error out=w425:errorcluster)  [unwired: 1 in, 5 out]
    n233 = Not Equal?(x=w429, y=w424) -> (x != y?=w428:bool)
    n234 = case shown="真" w428 {
      tunnel: [_ w431] -> _
      tunnel: w425 -> [_ _]
      frame False {
      }
      frame True {
        n235 = call "配置初始化.vi"() -> ("error out"=w431:errorcluster)  [unwired: 11 in]
      }
    }
    n236 = Wait (ms)(milliseconds to wait=u32 1000 ("等待时间（毫秒）")) -> ()  [unwired: 1 out]
  }
  n237 = flat-sequence {
    tunnel: w4 -> [_]
    frame #0 {
      n238 = control-ref of="周期设置"() -> (w436:refnum<vi>)
      n239 = call "New TimingControl.vi"("Reference"=w436) -> ("error out"=w434:errorcluster, "TimingControl out"=w435:refnum<class "TimingControl.lvclass">)  [unwired: 9 in]
      n240 = call "taskqueue ref.vi"() -> ("队列输出"=w438:refnum<queue>)  [unwired: 10 in, 1 out]
      n241 = while {
        tunnel: w438 -> [w456]
        shift-right: [w452] -> _
        shift-left: u32 0 ("等待时间（毫秒）") -> [w450]
        shift-right: [w440] -> w433
        shift-left: w435 -> [w445]
        shift-right: [w439] -> w432
        shift-left: w434 -> [w444]
        stop <- FALSE stop-if-true
        n242 = global read "VAR总磷总氮全局变量.vi" "状态告警区"() -> (w458:T6)
        n243 = Unbundle By Name(w458) -> ("工作状态"=w455:u16, "系统时间"=w442:timestamp)
        n244 = Quotient & Remainder(x=w450, y=u32 30) -> (x-y*floor(x/y)=w448:u32)  [unwired: 1 out]
        n245 = Equal To 0?(x=w448) -> (x = 0?=w447:bool)
        n246 = case shown="1, 默认" w455 {
          tunnel: [FALSE TRUE] -> w441
          frame 0 {
          }
          frame 1, Default {
          }
        }
        n247 = Increment(x=w450) -> (x+1=w454:u32)
        n248 = Wait (ms)(milliseconds to wait=u32 500 ("等待时间（毫秒）")) -> ()  [unwired: 1 out]
        n249 = property class="TimingControl"(reference=w445, error in=w444, "Properties:仪器时间"=w442, "Properties:仪器运行状态"=w441) -> (reference out=w440:refnum<class "TimingControl.lvclass">, error out=w439:errorcluster, "Properties:命令输出"=w443:cluster{"启动":bool, "控制命令":T12, "测量参数":T13})
        n250 = Unbundle By Name(w443) -> ("启动"=w451:bool, "控制命令"=w457:T12)
        n251 = And(x=w451, y=w447) -> (x .and. y?=w446:bool)
        n252 = Select(t=w454, s=w451, f=u32 0 ("等待时间（毫秒）")) -> (s? t:f=w452:u32)
        n253 = case shown="真" w446 {
          tunnel: w457 -> [_ w462]
          tunnel: w456 -> [_ w465]
          frame False {
          }
          frame True {
            n254 = Get Queue Status(queue=w465) -> (queue out=w463:refnum<queue>, # elements in queue=w464:i32)  [unwired: 2 in, 6 out]
            n255 = Equal To 0?(x=w464) -> (x = 0?=w461:bool)
            n256 = case shown="真" w461 {
              tunnel: w463 -> [_ w467]
              tunnel: w462 -> [_ w466]
              frame False {
              }
              frame True {
                n257 = Enqueue Element(queue=w467, element=w466) -> ()  [unwired: 2 in, 3 out]
              }
            }
          }
        }
      }
      n258 = call "试剂余量后台任务.vi"() -> ()  [unwired: 12 in]
      n259 = call "task.vi"() -> ()  [unwired: 12 in]
      n260 = call "更新调试流程.vi"() -> ()  [unwired: 12 in]
      n261 = call "Close TimingControl.vi"("error in (no error)"=w432, "TimingControl in"=w433) -> ()  [unwired: 9 in, 1 out]
    }
  }
  n262 = while {
    tunnel: w4 -> [_]
    stop <- FALSE stop-if-true
    n263 = flat-sequence {
      frame #0 {
        n264 = global read "model config var.vi" "启动队列名称"() -> (w471:cluster{"String":string, "Value":u16}[])
        n265 = for {
          tunnel: w471 -> [w479] mode=indexing
          shift-right: [w478] -> w474
          shift-left: "" -> [w477]
          tunnel: [w476] -> w472 mode=indexing
          n266 = Unbundle By Name(w479) -> ("String"=w476:string)
          n267 = Concatenate Strings(w477, w476) -> (w478:string)
        }
        n268 = global write "VAR总磷总氮全局变量.vi" "模块名称"(w474) -> ()
        n269 = property on="单选按钮" class="RadioBtnsControl (严格)"() -> ("Controls[]"=w473:refnum<vi>[])  [unwired: 2 in, 2 out]
        n270 = for {
          tunnel: w473 -> [w487] mode=indexing
          tunnel: w472 -> [w486]
          n271 = property class="Ctl"(reference=w487) -> (reference out=w485:refnum<vi>, "Label.Text"=w481:string)  [unwired: 1 in, 1 out]
          n272 = case shown="\"COD\"" w481 {
            selector: w481 -> [w488 _]
            tunnel: [w488 "CODcr"] -> w480
            frame Default {
            }
            frame "COD" {
            }
          }
          n273 = Search 1D Array(1D array=w486, element=w480) -> (index of element=w484:i32)  [unwired: 1 in]
          n274 = Not Equal?(x=w484, y=-1) -> (x != y?=w482:bool)
          n275 = property class="Ctl"(reference=w485, "Visible"=w482) -> ()  [unwired: 1 in, 2 out]
        }
      }
      frame #1 {
        n276 = Wait (ms)(milliseconds to wait=u32 1000 ("等待时间（毫秒）")) -> ()  [unwired: 1 out]
      }
    }
  }
  n277 = vi-ref "参数设置页.vi"() -> (w16:refnum<vi>)
  n278 = vi-ref "校准设置页.vi"() -> (w12:refnum<vi>)
  n279 = call "时间延迟"("error in (no error)"=w3) -> ("error out"=w26:errorcluster)  [unwired: 10 in]
  n280 = Obtain Notifier(name (unnamed)=w19, notification data type=FALSE) -> (notifier out=w20:refnum<notifier>)  [unwired: 2 in, 2 out]
  n281 = Obtain Queue(name (unnamed)=w19, element data type=cluster{"命令":string, "data":variant} {"命令"="", "data"=variant}) -> (queue out=w22:refnum<queue>)  [unwired: 3 in, 2 out]
  n282 = property class="VI"(reference=w16, error in=w8) -> (reference out=w14:refnum<vi>, "Exec.State"=w15:T14)  [unwired: 1 out]
  n283 = property class="VI"(reference=w12, error in=w7) -> (reference out=w10:refnum<vi>, "Exec.State"=w11:T14)  [unwired: 1 out]
  n284 = while {
    tunnel: w22 -> [w502]
    stop <- FALSE stop-if-true
    n285 = global read "总磷总氮断电保存全局变量.vi" "MB通信方式选择"() -> (w500:enum16{"串口", "TCP"})
    n286 = Get Queue Status(queue=w502) -> (queue out=w501:refnum<queue>, # elements in queue=w497:i32)  [unwired: 2 in, 6 out]
    n287 = global read "VAR总磷总氮全局变量.vi" "MB session in"() -> (w498:refnum<class "MB_Master.lvclass">)
    n288 = global read "VAR总磷总氮全局变量.vi" "升级固件关闭心跳包"() -> (w494:bool)
    n289 = Not(x=w494) -> (.not. x?=w493:bool)
    n290 = case shown="\"串口\", 默认" w500 {
      tunnel: [w505 w506] -> w499
      frame "串口", Default {
        n291 = global read "总磷总氮断电保存全局变量.vi" "VISA Resource"() -> (w505:refnum<visa-resource-name>)
      }
      frame "TCP" {
        n292 = global read "总磷总氮断电保存全局变量.vi" "IP"() -> (w506:string)
      }
    }
    "字符串 2" <- w499
    n293 = property class="MB_Master"(reference=w498) -> ("Properties:Session Valid"=w496:bool)  [unwired: 1 in, 2 out]
    n294 = Equal To 0?(x=w497) -> (x = 0?=w491:bool)
    n295 = Compound Arithmetic op=AND ("复合运算")(w496, w493) -> (w495:bool)
    n296 = global write "VAR总磷总氮全局变量.vi" "心跳包打开状态"(w495) -> ()
    n297 = And(x=w491, y=w495) -> (x .and. y?=w492:bool)
    n298 = case shown="真" w492 {
      tunnel: w501 -> [_ w529]
      frame False {
      }
      frame True {
        n299 = global read "VAR总磷总氮全局变量.vi" "状态告警区"() -> (w522:T6)
        n300 = global read "VAR总磷总氮全局变量.vi" "MB session in"() -> (w516:refnum<class "MB_Master.lvclass">)
        n301 = Unbundle By Name(w522) -> ("系统时间"=w509:timestamp, "工作状态"=w518:u16)
        n302 = property class="MB_Master"(reference=w516) -> ("Properties:Session Valid"=w514:bool)  [unwired: 1 in, 2 out]
        n303 = Get Date/Time In Seconds() -> (seconds since 1Jan1904=w528:timestamp)
        n304 = global read "VAR总磷总氮全局变量.vi" "通讯状态"() -> (w517:bool)
        n305 = case shown="真" w514 {
          tunnel: [_ w531] -> w513
          frame False {
          }
          frame True {
            n306 = global read "VAR总磷总氮全局变量.vi" "MB session in"() -> (w530:refnum<class "MB_Master.lvclass">)
            n307 = call "版本号读取.vi"("MB session in"=w530) -> ("error out"=w531:errorcluster, "固件版本号"=w532:string)  [unwired: 8 in, 1 out]
            "固件版本号" <- w532
            n308 = global write "VAR总磷总氮全局变量.vi" "固件版本号"(w532) -> ()
          }
        }
        n309 = Subtract(x=w528, y=w509) -> (x-y=w527:dbl)
        n310 = Not Equal?(x=w509, y=timestamp(0 s since 1904-01-01)) -> (x != y?=w507:bool)
        n311 = And(x=w514, y=w517) -> (x .and. y?=w515:bool)
        n312 = Absolute Value(x=w527) -> (abs(x)=w526:dbl)
        n313 = Greater Or Equal?(x=w526, y=30.0) -> (x >= y?=w524:bool)
        n314 = global read "VAR总磷总氮全局变量.vi" "通讯状态"() -> (w510:bool)
        n315 = Compound Arithmetic op=AND ("复合运算")(w524, w510, w507) -> (w519:bool)
        n316 = case shown="真" w515 {
          tunnel: [_ w533] -> w512
          tunnel: w513 -> [_ w534]
          frame False {
          }
          frame True {
            n317 = global read "VAR总磷总氮全局变量.vi" "MB session in"() -> (w536:refnum<class "MB_Master.lvclass">)
            n318 = call "序列号读取.vi"("Error in"=w534, "MB session in"=w536) -> ("error out"=w533:errorcluster, "序列号"=w535:string)  [unwired: 7 in, 1 out]
            n319 = global write "VAR总磷总氮全局变量.vi" "序列号"(w535) -> ()
          }
        }
        n320 = Unbundle By Name(w512) -> ("status"=w511:bool)
        n321 = global read "model config var.vi" "启动队列名称"() -> (w520:cluster{"String":string, "Value":u16}[])
        n322 = Not(x=w511) -> ()  [unwired: 1 out]
        n323 = for {
          tunnel: [w554] -> w521 mode=indexing
          tunnel: w520 -> [w555] mode=indexing
          tunnel: w512 -> [_]
          n324 = Unbundle By Name(w555) -> ("Value"=w554:u16)
        }
        n325 = for {
          tunnel: w518 -> [w540]
          shift-right: [w541] -> w523
          shift-left: w529 -> [w543]
          tunnel: w521 -> [w537] mode=indexing
          n326 = Equal?(x=w540, y=T15."空闲") -> (x = y?=w538:bool)
          n327 = Bundle By Name(cluster=cluster{"命令":string, "data":variant} {"命令"="", "data"=variant} ("元素"), "命令"="读状态告警区", "data"=w537) -> (w545:cluster{"命令":string, "data":variant})
          n328 = Enqueue Element(queue=w543, element=w545) -> (queue out=w542:refnum<queue>)  [unwired: 2 in, 2 out]
          n329 = case shown="真" w538 {
            tunnel: w542 -> [w547 w550]
            tunnel: w537 -> [_ w549]
            tunnel: [w547 w548] -> w541
            frame False {
            }
            frame True {
              n330 = Bundle By Name(cluster=cluster{"命令":string, "data":variant} {"命令"="", "data"=variant} ("元素"), "命令"="读测量数据区", "data"=w549) -> (w552:cluster{"命令":string, "data":variant})
              n331 = Enqueue Element(queue=w550, element=w552) -> (queue out=w548:refnum<queue>)  [unwired: 2 in, 2 out]
            }
          }
        }
        n332 = case shown="真" w519 {
          tunnel: w523 -> [_ w557]
          frame False {
          }
          frame True {
            n333 = call "总磷总氮启动命令.vi"("参数"=T16 {"站号"=3, "量程切换"=enum."AUTO", "控制命令"=enum."校时", "模式设置"=enum."待机", "测量间隔"=0}) -> ("启动命令"=w556:cluster{"命令":string, "data":variant})  [unwired: 10 in]
            n334 = Enqueue Element(queue=w557, element=w556) -> ()  [unwired: 2 in, 3 out]
          }
        }
      }
    }
    n335 = Wait (ms)(milliseconds to wait=u32 1000 ("等待时间（毫秒）")) -> ()  [unwired: 1 out]
  }
  n336 = while {
    tunnel: w26 -> [_]
    stop <- FALSE stop-if-true
    n337 = global read "VAR总磷总氮全局变量.vi" "状态告警区"() -> (w590:T6)
    n338 = global read "VAR总磷总氮全局变量.vi" "状态告警区"() -> (w588:T6)
    n339 = global read "VAR总磷总氮全局变量.vi" "状态告警区"() -> (w591:T6)
    n340 = global read "VAR总磷总氮全局变量.vi" "状态告警区"() -> (w592:T6)
    n341 = Unbundle By Name(w590) -> ("flowid"=w561:u16, "工作状态"=w580:u16, "id"=w581:u16)
    n342 = Unbundle By Name(w588) -> ("日志代码"=w587:u16)
    n343 = Unbundle By Name(w591) -> ("日志代码"=w564:u16)
    n344 = Unbundle By Name(w592) -> ("id"=w568:u16, "flowid"=w567:u16, "量程"=w566:u16, "工作状态"=w559:u16, "F0"=→"F0":sgl, "F1"=→"F1":sgl, "F2"=→"F2":sgl, "F3"=→"F3":sgl, "ADC"=→"ADC":sgl, "总磷控温温度1"=→"消解温度":sgl, "营养盐控温温度2"=→"注射器温度":sgl)
    n345 = Not Equal To 0?(x=w580) -> (x != 0?=w578:bool)
    n346 = case shown="0" w580 {
      frame 0 {
        n347 = local write "数组"(string[] [] ("数组")) -> ()
      }
      frame 1, Default {
      }
    }
    n348 = feedback #1(w587) -> (w589:u16)
    n349 = feedback-in #1(w587) -> ()
    n350 = feedback-in #2(w564) -> ()
    n351 = feedback #2(w564) -> (w594:u16)
    n352 = property on="总步数" class="DigNum (严格)"() -> ("Value"=w565:i32)  [unwired: 2 in, 2 out]
    n353 = Subtract(x=w564, y=1) -> (x-y=→"多列列表框":i32)
    n354 = Not Equal?(x=w587, y=w589) -> (x != y?=w586:bool)
    n355 = Not Equal?(x=w564, y=w594) -> (x != y?=w593:bool)
    n356 = Divide(x=w564, y=w565) -> (x/y=w563:dbl)
    n357 = Bundle("id"=w568, "flowid"=w567, "量程"=w566) -> (w569:cluster{"id":u16, "flowid":u16, "量程":u16})  [unwired: 1 in]
    n358 = call <vilib>:"Boolean Crossing PtByPt.vi"("direction"=enum16{"either", "false-true", "true-false"}."false-true", "input"=w578) -> ("crossing"=w582:bool)  [unwired: 1 in]
    n359 = call <vilib>:"Boolean Crossing PtByPt.vi"("direction"=enum16{"either", "false-true", "true-false"}."true-false", "input"=w578) -> ("crossing"=w577:bool)  [unwired: 1 in]
    n360 = case shown="真" w586 {
      frame False {
      }
      frame True {
        n361 = property on="多列列表框" class="MCListbox (严格)"() -> ("ItemNames"=w666:string[][], "Value"=w662:i32)  [unwired: 2 in, 2 out]
        n362 = Index Array(array=w666, index (row)=w662) -> (element=w665:string[])  [unwired: 1 in]
        n363 = Index Array(array=w665) -> (element=w664:string)  [unwired: 1 in]
        n364 = call "过滤筛选流程.vi"("字符串"=w664) -> ("匹配后偏移量"=w663:i32)  [unwired: 10 in]
        n365 = case shown="默认" w663 {
          tunnel: w664 -> [w668 _]
          tunnel: w662 -> [w667 _]
          frame Default {
            n366 = case shown="默认" w668 {
              selector: w668 -> [w674 w681]
              tunnel: [w674 w681] -> w670
              tunnel: [string[] [] ("数组") w676] -> w669
              tunnel: w667 -> [_ w680]
              frame "读数" {
              }
              frame Default {
                n367 = Equal?(x=w680, y=1) -> (x = y?=w678:bool)
                n368 = Select(t=string[] [], s=w678, f="数组") -> (s? t:f=w676:string[])
              }
            }
            n369 = for {
              N: 1 -> [_]
              tunnel: w670 -> [w683]
              shift-right: [w682] -> w671
              shift-left: w669 -> [w684]
              n370 = Search 1D Array(1D array=w684, element=w683) -> (index of element=w687:i32)  [unwired: 1 in]
              n371 = Format Into String(format string="%s" ("格式字符串"), w683) -> (resulting string=w688:string)  [unwired: 2 in, 1 out]
              n372 = Equal?(x=w687, y=-1) -> (x = y?=w685:bool)
              n373 = case shown="真" w685 {
                tunnel: w688 -> [_ w698]
                tunnel: w684 -> [w690 w702]
                tunnel: w683 -> [_ w701]
                tunnel: [w690 w700] -> w682
                frame False {
                }
                frame True {
                  n374 = global read "VAR总磷总氮全局变量.vi" "状态告警区"() -> (w697:T6)
                  n375 = global read "VAR总磷总氮全局变量.vi" "状态告警区"() -> (w712:T6)
                  n376 = global read "VAR总磷总氮全局变量.vi" "状态告警区"() -> (w715:T6)
                  n377 = Insert Into Array(array=w702, new element=w701) -> (w700:string[])  [unwired: 1 in]
                  n378 = Unbundle By Name(w697) -> ("工作状态"=w696:u16, "flowid"=w691:u16)
                  n379 = Unbundle By Name(w712) -> ("F0"=w709:sgl, "F1"=w708:sgl, "F2"=w707:sgl, "F3"=w706:sgl, "id"=w705:u16, "flowid"=w704:u16, "量程"=w703:u16)
                  n380 = Unbundle By Name(w715) -> ("id"=w693:u16)
                  n381 = case shown="2" w696 {
                    selector: w696 -> [w717 _ _ _ _ _ _ _ _ _ _ _]
                    tunnel: [w716 "【水样测试】" ("字符串") w720 "【零点核查】" ("字符串") "【跨度核查】" ("字符串") "【空白测试】" ("字符串") "【平行样测试】" ("字符串") "【加标回收】" ("字符串") "【空白校准】" ("字符串") "【标样校准】" ("字符串") "【单步调试】" ("字符串") w731] -> w694
                    tunnel: w691 -> [_ _ w719 _ _ _ _ _ _ _ _ _]
                    frame 0, Default {
                      n382 = Number To Decimal String(number=w717) -> (decimal integer string=w716:string)  [unwired: 1 in]
                    }
                    frame 1 {
                    }
                    frame 2 {
                      n383 = case shown="5" w719 {
                        tunnel: ["【标样核查】" ("字符串") "【快捷测试】" ("字符串")] -> w720
                        frame Default {
                        }
                        frame 5 {
                        }
                      }
                    }
                    frame 3 {
                    }
                    frame 4 {
                    }
                    frame 5 {
                    }
                    frame 6 {
                    }
                    frame 7 {
                    }
                    frame 8 {
                    }
                    frame 9 {
                    }
                    frame 254 {
                    }
                    frame 255 {
                      n384 = local read "简易步骤名称"() -> (w733:string)
                      n385 = Format Into String(format string="(%s)" ("格式字符串"), initial string="【简易流程】" ("工作状态"), w733) -> (resulting string=w731:string)  [unwired: 1 in, 1 out]
                    }
                  }
                  n386 = call "id参数转换.vi"("id"=w693) -> ("table输出"=w692:string)  [unwired: 9 in, 1 out]
                  n387 = Format Into String(format string="F0=%#f,F1=%#f,F2=%#f,F3=%#f,Flow=%d-%-d-%-d" ("格式字符串"), w709, w708, w707, w706, w705, w704, w703) -> (resulting string=w710:string)  [unwired: 2 in, 1 out]
                  n388 = Concatenate Strings(w694, w698) -> (w695:string)
                  n389 = Get Date/Time In Seconds() -> (seconds since 1Jan1904=w713:timestamp)
                  n390 = Bundle By Name(cluster=T17 {"时间标识"=timestamp(0 s since 1904-01-01), "设备"="", "日志信息"="", "流程参数"=""} ("data in"), "时间标识"=w713, "设备"=w692, "日志信息"=w695, "流程参数"=w710) -> (w714:T17)
                  n391 = call "总磷总氮操作日志.vi"("data in"=w714) -> ()  [unwired: 10 in, 1 out]
                }
              }
            }
            n392 = local write "数组"(w671) -> ()
          }
          frame -1 {
          }
        }
      }
    }
    n393 = case shown="真" w593 {
      tunnel: w564 -> [_ w768]
      frame False {
      }
      frame True {
        n394 = Subtract(x=w768, y=1) -> (x-y=w766:i32)
        n395 = Subtract(x=w766, y=5) -> (x-y=w770:i32)
        n396 = Greater Or Equal To 0?(x=w770) -> (x >= 0?=w769:bool)
        n397 = property on="多列列表框" class="MCListbox (严格)"() -> (error out=w774:errorcluster, "TopLeft"=w775:T18)  [unwired: 2 in, 1 out]
        n398 = Select(t=w770, s=w769, f=0) -> (s? t:f=w771:i32)
        n399 = Bundle By Name(cluster=w775, "Row"=w771) -> (w776:T18)
        n400 = property on="多列列表框" class="MCListbox (严格)"(error in=w774, "TopLeft"=w776) -> ()  [unwired: 1 in, 2 out]
      }
    }
    n401 = while {
      tunnel: w569 -> [w750]
      shift-right: [w746] -> _
      shift-left: _ -> [w747]
      shift-right: [w739] -> _
      shift-left: _ -> [w748]
      shift-right: [w740] -> _
      shift-left: _ -> [w745]
      shift-right: [w736] -> _
      shift-left: _ -> [w743]
      tunnel: w559 -> [w736]
      stop <- TRUE stop-if-true
      n402 = Not Equal?(x=w743, y=w736) -> (x != y?=w742:bool)
      n403 = case shown="255" w736 {
        tunnel: [w751 w752] -> w740
        frame 0, Default {
          n404 = global read "总磷总氮断电保存全局变量.vi" "流程路径"() -> (w751:path)
        }
        frame 255 {
          n405 = global read "总磷总氮断电保存全局变量.vi" "简易流程路径"() -> (w752:path)
        }
      }
      n406 = Not Equal To 0?(x=w736) -> (x != 0?=w735:bool)
      n407 = Not Equal?(x=w745, y=w740) -> (x != y?=w741:bool)
      n408 = Compound Arithmetic op=OR ("复合运算")(w741, w742) -> (w744:bool)
      n409 = And(x=w735, y=w744) -> (x .and. y?=w737:bool)
      n410 = case shown="真" w737 {
        tunnel: [w754 w764] -> w739
        tunnel: [w753 w763] -> w746
        tunnel: w750 -> [_ w758]
        tunnel: w748 -> [w754 _]
        tunnel: w747 -> [w753 _]
        tunnel: w740 -> [_ w757]
        tunnel: w736 -> [_ w756]
        frame False {
        }
        frame True {
          n411 = call "斯坦道XML解析.vi"("工作状态"=w756, "添加的路径"=w757, "参数簇"=w758) -> ("简易步骤名称"=→"简易步骤名称":string, "步骤时间"=w759:string[], "步骤名"=w761:string[])  [unwired: 6 in]
          n412 = for {
            tunnel: w761 -> [_] mode=indexing
            tunnel: [w765] -> w762 mode=indexing
            i -> [w765]
          }
          n413 = Build Array(w761, w759) -> (w760:string[][])
          n414 = Transpose 2D Array(2D array=w760) -> (transposed array=w763:string[][])
          n415 = Number To Decimal String(number=w762) -> (decimal integer string=w764:string[])  [unwired: 1 in]
        }
      }
      n416 = property on="多列列表框" class="MCListbox (严格)"("ItemNames"=w746, "RowHdrs[]"=w739) -> ()  [unwired: 2 in, 2 out]
      n417 = Array Size(array=w739) -> (size(s)=→"总步数":i32)
    }
    n418 = Multiply(x=w563, y=100.0) -> (x*y=w560:dbl)
    "滑动杆" <- w560
    n419 = case shown="真" w582 {
      tunnel: w580 -> [_ w639]
      tunnel: w581 -> [_ w636]
      tunnel: w561 -> [_ w634]
      frame False {
      }
      frame True {
        n420 = case shown="8" w639 {
          selector: w639 -> [w646 _ _ _ _ _ _ _ _ _ _ _]
          tunnel: [w645 "【水样测试】" ("字符串") w649 "【零点核查】" ("字符串") "【跨度核查】" ("字符串") "【空白测试】" ("字符串") "【平行样测试】" ("字符串") "【加标回收】" ("字符串") "【空白校准】" ("字符串") "【标样校准】" ("字符串") "【单步调试】" ("字符串") "【简易流程】" ("字符串")] -> w644
          tunnel: w634 -> [_ _ w648 _ _ _ _ _ _ _ _ _]
          frame 0, Default {
            n421 = Number To Decimal String(number=w646) -> (decimal integer string=w645:string)  [unwired: 1 in]
          }
          frame 1 {
          }
          frame 2 {
            n422 = case shown="5" w648 {
              tunnel: ["【标样核查】" ("字符串") "【快捷测试】" ("字符串")] -> w649
              frame 0, Default {
              }
              frame 5 {
              }
            }
          }
          frame 3 {
          }
          frame 4 {
          }
          frame 5 {
          }
          frame 6 {
          }
          frame 7 {
          }
          frame 8 {
          }
          frame 9 {
          }
          frame 254 {
          }
          frame 255 {
          }
        }
        n423 = call "id参数转换.vi"("id"=w636) -> ("table输出"=w635:string)  [unwired: 9 in, 1 out]
        n424 = Concatenate Strings("<<" ("字符串"), w644, "启动" ("字符串")) -> (w643:string)
        n425 = Get Date/Time In Seconds() -> (seconds since 1Jan1904=w641:timestamp)
        n426 = Bundle By Name(cluster=T17 {"时间标识"=timestamp(0 s since 1904-01-01), "设备"="", "日志信息"="", "流程参数"=""} ("data in"), "时间标识"=w641, "设备"=w635, "日志信息"=w643) -> (w640:T17)
        n427 = call "总磷总氮操作日志.vi"("data in"=w640) -> ()  [unwired: 10 in, 1 out]
      }
    }
    n428 = case shown="真" w577 {
      tunnel: w581 -> [_ w612]
      tunnel: w561 -> [_ w598]
      frame False {
      }
      frame True {
        n429 = global read "VAR总磷总氮全局变量.vi" "最近一次工作状态"() -> (w597:u16)
        n430 = global read "VAR总磷总氮全局变量.vi" "状态告警区"() -> (w610:T6)
        n431 = call "id参数转换.vi"("id"=w612) -> ("table输出"=w611:string)  [unwired: 9 in, 1 out]
        n432 = case shown="2" w597 {
          selector: w597 -> [w619 _ _ _ _ _ _ _ _ _ _ _]
          tunnel: [w618 "【水样测试】" ("字符串") w622 "【零点核查】" ("字符串") "【跨度核查】" ("字符串") "【空白测试】" ("字符串") "【平行样测试】" ("字符串") "【加标回收】" ("字符串") "【空白校准】" ("字符串") "【标样校准】" ("字符串") "【单步调试】" ("字符串") "【简易流程】" ("字符串")] -> w600
          tunnel: w598 -> [_ _ w621 _ _ _ _ _ _ _ _ _]
          frame 0, Default {
            n433 = Number To Decimal String(number=w619) -> (decimal integer string=w618:string)  [unwired: 1 in]
          }
          frame 1 {
          }
          frame 2 {
            n434 = case shown="0, 默认" w621 {
              tunnel: ["【标样核查】" ("字符串") "【快捷测试】" ("字符串")] -> w622
              frame 0, Default {
              }
              frame 5 {
              }
            }
          }
          frame 3 {
          }
          frame 4 {
          }
          frame 5 {
          }
          frame 6 {
          }
          frame 7 {
          }
          frame 8 {
          }
          frame 9 {
          }
          frame 254 {
          }
          frame 255 {
          }
        }
        n435 = Unbundle By Name(w610) -> ("F0"=w609:sgl, "F1"=w608:sgl, "F2"=w607:sgl, "F3"=w606:sgl, "id"=w605:u16, "flowid"=w604:u16, "量程"=w603:u16)
        n436 = Format Into String(format string="F0=%#f,F1=%#f,F2=%#f,F3=%#f,Flow=%d-%-d-%-d" ("格式字符串"), w609, w608, w607, w606, w605, w604, w603) -> (resulting string=w601:string)  [unwired: 2 in, 1 out]
        n437 = Concatenate Strings(w600, "停止" ("字符串"), ">>" ("字符串")) -> (w617:string)
        n438 = Get Date/Time In Seconds() -> (seconds since 1Jan1904=w615:timestamp)
        n439 = Bundle By Name(cluster=T17 {"时间标识"=timestamp(0 s since 1904-01-01), "设备"="", "日志信息"="", "流程参数"=""} ("data in"), "时间标识"=w615, "设备"=w611, "日志信息"=w617, "流程参数"=w601) -> (w614:T17)
        n440 = call "总磷总氮操作日志.vi"("data in"=w614) -> ()  [unwired: 10 in, 1 out]
      }
    }
    n441 = global write "VAR总磷总氮全局变量.vi" "测试进度"(w560) -> ()
    n442 = Wait (ms)(milliseconds to wait=u32 1000 ("等待时间（毫秒）")) -> ()  [unwired: 1 out]
  }
  n443 = case shown="\"Bad\", 默认" w15 {
    tunnel: w14 -> [w777 w781]
    tunnel: [w777 w778] -> w13
    frame "Bad", Default {
    }
    frame "Idle" {
      n444 = invoke class="VI" method="Run VI"(reference=w781, "Wait until done"=FALSE ("结束前等待"), "Auto Dispose Ref"=TRUE ("自动销毁引用")) -> (reference out=w778:refnum<vi>)  [unwired: 2 in, 4 out]
    }
  }
  n445 = case shown="\"Bad\", 默认" w11 {
    tunnel: w10 -> [w782 w786]
    tunnel: [w782 w783] -> w9
    frame "Bad", Default {
    }
    frame "Idle" {
      n446 = invoke class="VI" method="Run VI"(reference=w786, "Wait until done"=FALSE ("结束前等待"), "Auto Dispose Ref"=TRUE ("自动销毁引用")) -> (reference out=w783:refnum<vi>)  [unwired: 2 in, 4 out]
    }
  }
  n447 = while {
    tunnel: w22 -> [w790]
    tunnel: w20 -> [w789]
    tunnel: w13 -> [w788]
    tunnel: w9 -> [w787]
    stop <- FALSE stop-if-true
    n448 = event shown="[9] \"调试\": 值改变" {
      selector: _ -> [_ _ _ _ _ _ _ _ _ _ _ _ _ _]
      dyn-events: _ -> [_ _ _ _ _ _ _ _ _ _ _ _ _ _]
      timeout: _ -> [_ _ _ _ _ _ _ _ _ _ _ _ _ _]
      tunnel: w790 -> [_ _ _ _ _ _ _ _ w804 _ w823 _ _ _]
      tunnel: w789 -> [_ _ _ _ _ _ _ _ _ _ w822 _ _ _]
      tunnel: w788 -> [_ _ _ _ _ _ _ _ _ _ _ w827 _ _]
      tunnel: w787 -> [_ _ _ _ _ _ _ _ _ _ _ _ w833 _]
      event Timeout {
        n449 = event-data() -> ()  [unwired: 1 in, 3 out]
      }
      event "流程操作": Value Change {
        n450 = event-data() -> ()  [unwired: 1 in, 6 out]
        n451 = global read "总磷总氮断电保存全局变量.vi" "流程路径"() -> (w793:path)
        n452 = global read "总磷总氮断电保存全局变量.vi" "简易流程路径"() -> (w792:path)
        n453 = call "流程批量写入.vi"("简易流程路径"=w792, "添加的路径"=w793) -> ()  [unwired: 10 in]
      }
      event "温度曲线": Value Change {
        n454 = event-data() -> ()  [unwired: 1 in, 6 out]
        n455 = call "温度曲线显示.vi"() -> ()  [unwired: 12 in]
      }
      event "试剂余量": Value Change {
        n456 = event-data() -> ()  [unwired: 1 in, 6 out]
        n457 = call "试剂余量显示UI.vi"() -> ()  [unwired: 12 in]
      }
      event "灯值调整": Value Change {
        n458 = event-data() -> ()  [unwired: 1 in, 6 out]
        n459 = call "灯值调整对话框.vi"() -> ()  [unwired: 12 in]
      }
      event "布尔": Value Change {
        n460 = event-data() -> ("NewVal"=w794:bool)  [unwired: 1 in, 5 out]
        n461 = case shown="假" w794 {
          frame False {
            n462 = global write "VAR总磷总氮全局变量.vi" "权限等级"(enum16{"一级权限", "二级权限", "三级权限", "超级权限"}."一级权限" ("权限等级")) -> ()
          }
          frame True {
            n463 = global read "VAR总磷总氮全局变量.vi" "权限密码"() -> (w798:u32[])
            n464 = global read "VAR总磷总氮全局变量.vi" "权限等级"() -> (w796:enum16{"一级权限", "二级权限", "三级权限", "超级权限"})
            n465 = call "密码权限设置.vi"("权限输入"=w796, "权限密码"=w798) -> ("权限输出"=w797:enum16{"一级权限", "二级权限", "三级权限", "超级权限"})  [unwired: 9 in]
            n466 = global write "VAR总磷总氮全局变量.vi" "权限等级"(w797) -> ()
          }
        }
      }
      event "权限等级": Mouse Down {
        n467 = event-data() -> ()  [unwired: 1 in, 8 out]
        n468 = global read "VAR总磷总氮全局变量.vi" "权限密码"() -> (w801:u32[])
        n469 = global read "VAR总磷总氮全局变量.vi" "权限等级"() -> (w799:enum16{"一级权限", "二级权限", "三级权限", "超级权限"})
        n470 = call "密码权限设置.vi"("权限输入"=w799, "权限密码"=w801) -> ("权限输出"=w800:enum16{"一级权限", "二级权限", "三级权限", "超级权限"})  [unwired: 9 in]
        n471 = global write "VAR总磷总氮全局变量.vi" "权限等级"(w800) -> ()
      }
      event "外设固件": Value Change {
        n472 = event-data() -> ()  [unwired: 1 in, 6 out]
        n473 = call "流程固件设置对话框.vi"() -> ()  [unwired: 12 in]
      }
      event "手动启动": Value Change {
        n474 = event-data() -> ()  [unwired: 1 in, 6 out]
        n475 = call "总磷总氮启动参数对话框.vi"() -> ("确认"=w802:bool, "元素"=w803:cluster{"命令":string, "data":variant})  [unwired: 10 in]
        n476 = case shown="真" w802 {
          tunnel: w804 -> [_ w807]
          tunnel: w803 -> [_ w806]
          frame False {
          }
          frame True {
            n477 = Flush Queue(queue=w807) -> (queue out=w805:refnum<queue>)  [unwired: 1 in, 2 out]
            n478 = Enqueue Element(queue=w805, element=w806) -> ()  [unwired: 2 in, 3 out]
          }
        }
      }
      event "调试": Value Change {
        n479 = event-data() -> ()  [unwired: 1 in, 6 out]
        n480 = call "简易流程调试界面.vi"() -> ()  [unwired: 12 in]
      }
      event "停止": Value Change {
        n481 = event-data() -> ()  [unwired: 1 in, 6 out]
        n482 = global read "VAR总磷总氮全局变量.vi" "状态告警区"() -> (w809:T6)
        n483 = global read "VAR总磷总氮全局变量.vi" "状态告警区"() -> (w817:T6)
        n484 = Send Notification(notification=TRUE ("通知"), notifier=w822) -> ()  [unwired: 1 in, 2 out]
        n485 = Unbundle By Name(w809) -> ("id"=w808:u16)
        n486 = Unbundle By Name(w817) -> ("id"=w816:u16)
        n487 = call "id参数转换.vi"("id"=w808) -> ("table输出"=w810:string)  [unwired: 9 in, 1 out]
        n488 = Bundle By Name(cluster=T16 {"站号"=1, "量程切换"=enum."AUTO", "控制命令"=enum."停止测试", "模式设置"=enum."待机", "测量间隔"=0} ("参数"), "站号"=w816) -> (w818:T16)
        n489 = Get Date/Time In Seconds() -> (seconds since 1Jan1904=w813:timestamp)
        n490 = call "总磷总氮启动命令.vi"("参数"=w818) -> ("启动命令"=w819:cluster{"命令":string, "data":variant})  [unwired: 10 in]
        n491 = Bundle By Name(cluster=T19 {"时间"=timestamp(0 s since 1904-01-01), "参数"="", "日志信息"="", "流程参数"=""} ("data in"), "时间"=w813, "参数"=w810, "日志信息"="手动停止") -> (w814:T19)
        n492 = Enqueue Element(queue=w823, element=w819) -> (error out=w811:errorcluster)  [unwired: 2 in, 2 out]
        n493 = call "总磷总氮操作日志.vi"("错误输入（无错误）"=w811, "data in"=w814) -> ()  [unwired: 9 in, 1 out]
      }
      event "参数设置", "参数查询": Value Change {
        n494 = event-data() -> ()  [unwired: 1 in, 6 out]
        n495 = invoke on="子面板" class="SubPnl" method="Remove VI"() -> (error out=w828:errorcluster)  [unwired: 3 in, 2 out]
        n496 = global write "VAR总磷总氮全局变量.vi" "页面"(enum16{"主页", "参数页", "校准页"}."参数页" ("页面")) -> ()
        n497 = property on="仪器校准" class="Bool"("Visible"=TRUE ("可见")) -> ()  [unwired: 2 in, 2 out]
        n498 = property on="参数查询" class="Bool"("Visible"=FALSE ("可见")) -> ()  [unwired: 2 in, 2 out]
        n499 = invoke on="子面板" class="SubPnl" method="Insert VI"(error in=w828, "VI Ref"=w827) -> ()  [unwired: 2 in, 4 out]
        n500 = property on="窗格" class="Pane"("Origin"=T5 {"Horizontal"=0, "Vertical"=640} ("原点")) -> ()  [unwired: 2 in, 2 out]
      }
      event "仪器校准": Value Change {
        n501 = event-data() -> ()  [unwired: 1 in, 6 out]
        n502 = invoke on="子面板" class="SubPnl" method="Remove VI"() -> (error out=w834:errorcluster)  [unwired: 3 in, 2 out]
        n503 = global write "VAR总磷总氮全局变量.vi" "页面"(enum16{"主页", "参数页", "校准页"}."校准页" ("页面")) -> ()
        n504 = property on="仪器校准" class="Bool"("Visible"=FALSE ("可见")) -> ()  [unwired: 2 in, 2 out]
        n505 = invoke on="子面板" class="SubPnl" method="Insert VI"(error in=w834, "VI Ref"=w833) -> ()  [unwired: 2 in, 4 out]
        n506 = property on="参数查询" class="Bool"("Visible"=TRUE ("可见")) -> ()  [unwired: 2 in, 2 out]
      }
      event "返回": Value Change {
        n507 = event-data() -> ()  [unwired: 1 in, 6 out]
        n508 = global write "VAR总磷总氮全局变量.vi" "页面"(enum16{"主页", "参数页", "校准页"}."主页" ("页面")) -> ()
        n509 = property on="窗格" class="Pane"("Origin"=T5 {"Horizontal"=0, "Vertical"=0} ("原点")) -> ()  [unwired: 2 in, 2 out]
      }
    }
  }
